vi "Initialize.vi"(8 "error in (no error)":errorcluster, 10 "Opciones puerto":T1={"baud rate"=9600, "data bits"=8, "parity"=enum."None"} {"data bits" min=5 max=8 step=1}, 11 "Puerto Serial":refnum<visa-resource-name>) -> (0 "error out":errorcluster, 2 "Connected?":bool, 3 "VISA resource name out":refnum<visa-resource-name>)   [LabVIEW 2020, in "Control de MaP.lvlib"]
doc: "Establece la comunicación con el instrumento"
uses:
  Control de MaP.lvlib
  <vilib>/Instr/_visa.llb/VISA Set IO Buffer Mask.ctl
  <vilib>/Instr/_visa.llb/VISA Flush IO Buffer Mask.ctl
  <vilib>/Instr/_visa.llb/VISA Configure Serial Port (Instr).vi
  Controls/Com Port Options.ctl
  Arduino-Adafruit stepper/Arduino-Adafruit stepper.lvlib
panel:
  # "Centro de investigaciones en óptica.  ALL RIGHTS RESERVED."
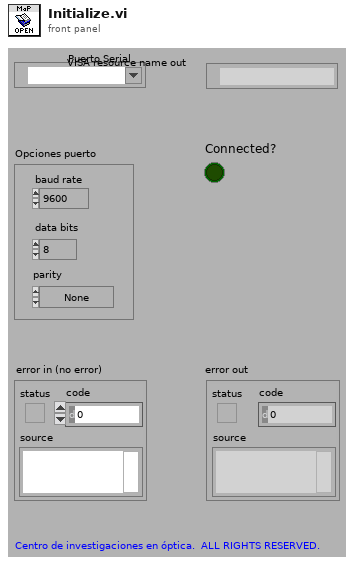
[diagram p1: front panel]
types:
  T1 = typedef "Arduino-Adafruit stepper.lvlib/Com Port Options.ctl" = cluster{"baud rate":u32, "data bits":u16, "parity":enum16{"None", "Odd", "Even", "Mark", "Space"}}
  T2 = typedef "VISA Set IO Buffer Mask.ctl" = u16
  T3 = typedef "VISA Flush IO Buffer Mask.ctl" = u16
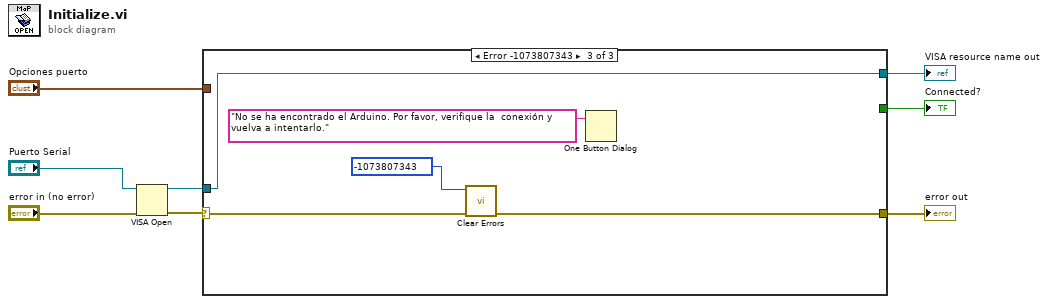
[diagram p0: block diagram]
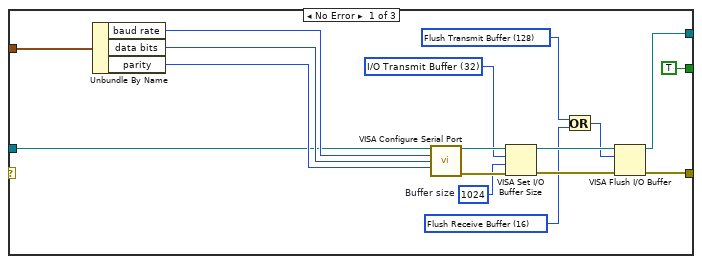
[diagram p2: hidden frame]
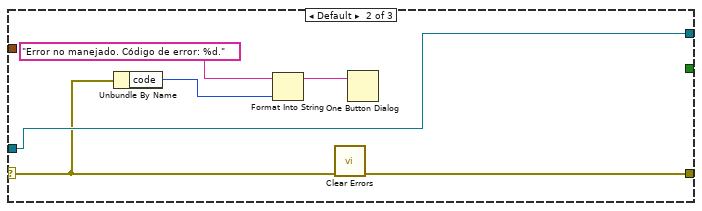
[diagram p3: hidden frame]
diagram:
  n1 = VISA Open(error in (no error)="error in (no error)", VISA resource name="Puerto Serial") -> (VISA resource name=w5:refnum<visa-resource-name>, error out=w3:errorcluster)  [unwired: 3 in]
  n2 = case shown="Error -1073807343" w3 {
    selector: w3 -> [_ w29 w34]
    tunnel: [w20 w31 w36] -> w8
    tunnel: [w21 w30 w32] -> w7
    tunnel: "Opciones puerto" -> [w25 _ _]
    tunnel: w5 -> [w10 w31 w36]
    tunnel: [TRUE _ _] -> w1
    frame No Error {
      w11 = u32 1024  # Buffer size
      w12 = T2 32 items=["I/O Receive Buffer"=16, "I/O Transmit Buffer"=32, "I/O Receive and Transmit Buffer"=48] ("Mask")
      w13 = T3 16 items=["Flush Receive Buffer"=16, "Write Transmit Buffer to Device"=32, "Flush Receive Buffer (No I/O)"=64, "Flush Transmit Buffer"=128] ("Mask")
      w15 = T3 128 items=["Flush Receive Buffer"=16, "Write Transmit Buffer to Device"=32, "Flush Receive Buffer (No I/O)"=64, "Flush Transmit Buffer"=128] ("Mask")
      n3 = Unbundle By Name(w25) -> ("baud rate"=w24:u32, "data bits"=w23:u16, "parity"=w22:enum16{"None", "Odd", "Even", "Mark", "Space"})
      n4 = call-poly "VISA Configure Serial Port"("VISA resource name"=w10, "baud rate (9600)"=w24, "data bits (8)"=w23, "parity (0:none)"=w22) -> ("VISA resource name out"=w19:refnum<visa-resource-name>, "error out"=w17:errorcluster)  [unwired: 10 in]
      n5 = VISA Set I/O Buffer Size(VISA resource name=w19, mask (16)=w12, size (4096)=w11, error in (no error)=w17) -> (VISA resource name out=w18:refnum<visa-resource-name>, error out=w16:errorcluster)
      n6 = Or(x=w15, y=w13) -> (x .or. y?=w14:T3)
      n7 = VISA Flush I/O Buffer(VISA resource name=w18, mask (16)=w14, error in (no error)=w16) -> (VISA resource name out=w20:refnum<visa-resource-name>, error out=w21:errorcluster)
    }
    frame Default {
      n8 = Unbundle By Name(w29) -> ("code"=w27:i32)
      n9 = Format Into String(initial string="Error no manejado. Código de error: %d.", w27) -> (resulting string=w26:string)  [unwired: 2 in, 1 out]
      n10 = call <vilib>:"Clear Errors.vi"("error in (no error)"=w29) -> ("error out"=w30:errorcluster)  [unwired: 5 in, 1 out]
      n11 = One Button Dialog(message=w26) -> ()  [unwired: 1 in, 1 out]
    }
    frame Error {
      n12 = call <vilib>:"Clear Errors.vi"("error in (no error)"=w34, "specific error code to clear (0: all)"=-1073807343) -> ("error out"=w32:errorcluster)  [unwired: 4 in, 1 out]
      n13 = One Button Dialog(message="No se ha encontrado el Arduino. Por favor, verifique la  conexión y vuelva a intentarlo.") -> ()  [unwired: 1 in, 1 out]
    }
  }
  "VISA resource name out" <- w8
  "error out" <- w7
  "Connected?" <- w1
